vi "Main.vi"(11 "Module Admin":refnum<class "Delacor_lib_QMH_Module Admin.lvclass">) -> ()   [LabVIEW 2019, in "CONFIG .lvlib"]
doc: "This template is based off of the Queued Message Handler design pattern and the Queued Message Handler project template that ships with LabVIEW.\n\nThe main difference is that the queue is private to this module and communication between modules is performed via Broadcast and Request events.\n\nRequest events are wrapped in public API methods and are handled in the Event Handling Loop (EHL) of this VI. Any module can register for Broadcast events sent by this module. The EHL generates messages based on user interface actions.\n\nThe Message Handling Loop (MHL) processes messages generated by the EHL, or by other messages. The messages are string values, so new messages can be added easily to the Message Cases case structure in the MHL. Each message cluster can also provide an optional value for Message Data, which is a variant that can be converted to whatever message-specific data is required.\n_____\nBased on Delacor QMH Project Template 5.0.0.82."
uses:
  CONFIG .lvlib
  <vilib>/Delacor/Delacor QMH/Libraries/Module Admin_class/Delacor_lib_QMH_Module Admin.lvclass
  Module Data--cluster.ctl
  STOP HELPER LOOP CONFIG Argument--cluster.ctl
  <vilib>/Delacor/Delacor QMH/Libraries/Message Queue_class/Delacor_lib_QMH_Message Queue.lvclass/Delacor_lib_QMH_Message Queue.ctl
  Stop Argument--cluster.ctl
  <vilib>/Delacor/Delacor QMH/Libraries/Module Admin_class/Delacor_lib_QMH_Module Admin.lvclass/Delacor_lib_QMH_Module Admin.ctl
  CONFIG START HELPER LOOP Argument--cluster.ctl
  <vilib>/Utility/miscctls.llb/LVPointTypeDef.ctl
  <vilib>/Delacor/Delacor QMH/Libraries/Message Queue_class/Delacor_lib_QMH_Enqueue Message (Single).vi
  <vilib>/Delacor/Delacor QMH/Libraries/Module Admin_class/Delacor_lib_QMH_Get External Launch.vi
  <vilib>/Utility/error.llb/Error Cluster From Error Code.vi
  <vilib>/ErrorRing/Error Ring.xnode
  <vilib>/Delacor/Delacor QMH/Libraries/Message Queue_class/Delacor_lib_QMH_Message Queue.lvclass
panel:
  in  "Simulate MHL Error":bool
  in  "Simulate EHL Error":bool
  out "error out":errorcluster
  out "Status":string
  # "Other QMH Modules communicate with this Module via its Public API (wrappers for its Request Events).\n\nThis Module communicates with other Modules via its Broadcast Events.\nAny module that wants to get these messages, just registers for this module's Broadcast events."
  # "This template is for the Delacor Modified Queued Message Handler design pattern.\n\nSee the block diagram for more information on how to use this template."
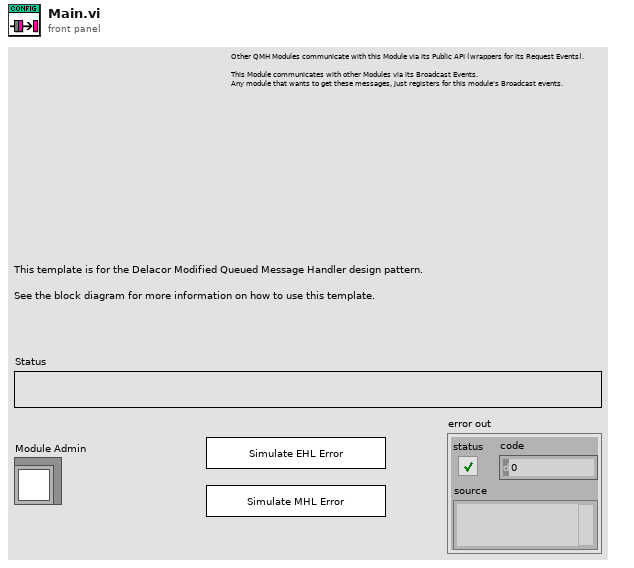
[diagram p1: front panel]
types:
  T1 = typedef "CONFIG .lvlib/Request Events--cluster.ctl" = cluster{"Stop Module":refnum<user-event>, "Show Panel":refnum<user-event>, "Hide Panel":refnum<user-event>, "Get Module Execution Status":refnum<user-event>, "Show Diagram":refnum<user-event>, "CONFIG START HELPER LOOP":refnum<user-event>, "STOP HELPER LOOP CONFIG":refnum<user-event>}
  T2 = typedef "CONFIG .lvlib/Module Data--cluster.ctl" = cluster{"Status":string}
  T3 = typedef "CONFIG .lvlib/STOP HELPER LOOP CONFIG Argument--cluster.ctl" = cluster{"Boolean":bool}
  T4 = enum32{"invalid lock state", "Not Locked", "Locked (No Password)", "Password-protected"}
  T5 = typedef "CONFIG .lvlib/Stop Argument--cluster.ctl" = cluster{"Origin":string, "Exit via Stop Module Req?":bool, "Wait for Module to stop?":bool}
  T6 = typedef "CONFIG .lvlib/CONFIG START HELPER LOOP Argument--cluster.ctl" = cluster{"DELAY TIMEOUT":i32}
  T7 = typedef "LVPointTypeDef.ctl" = cluster{"Horizontal":i16, "Vertical":i16}
  T8 = enum32{"Invalid", "Standard", "Closed", "Hidden", "Minimized", "Maximized"}
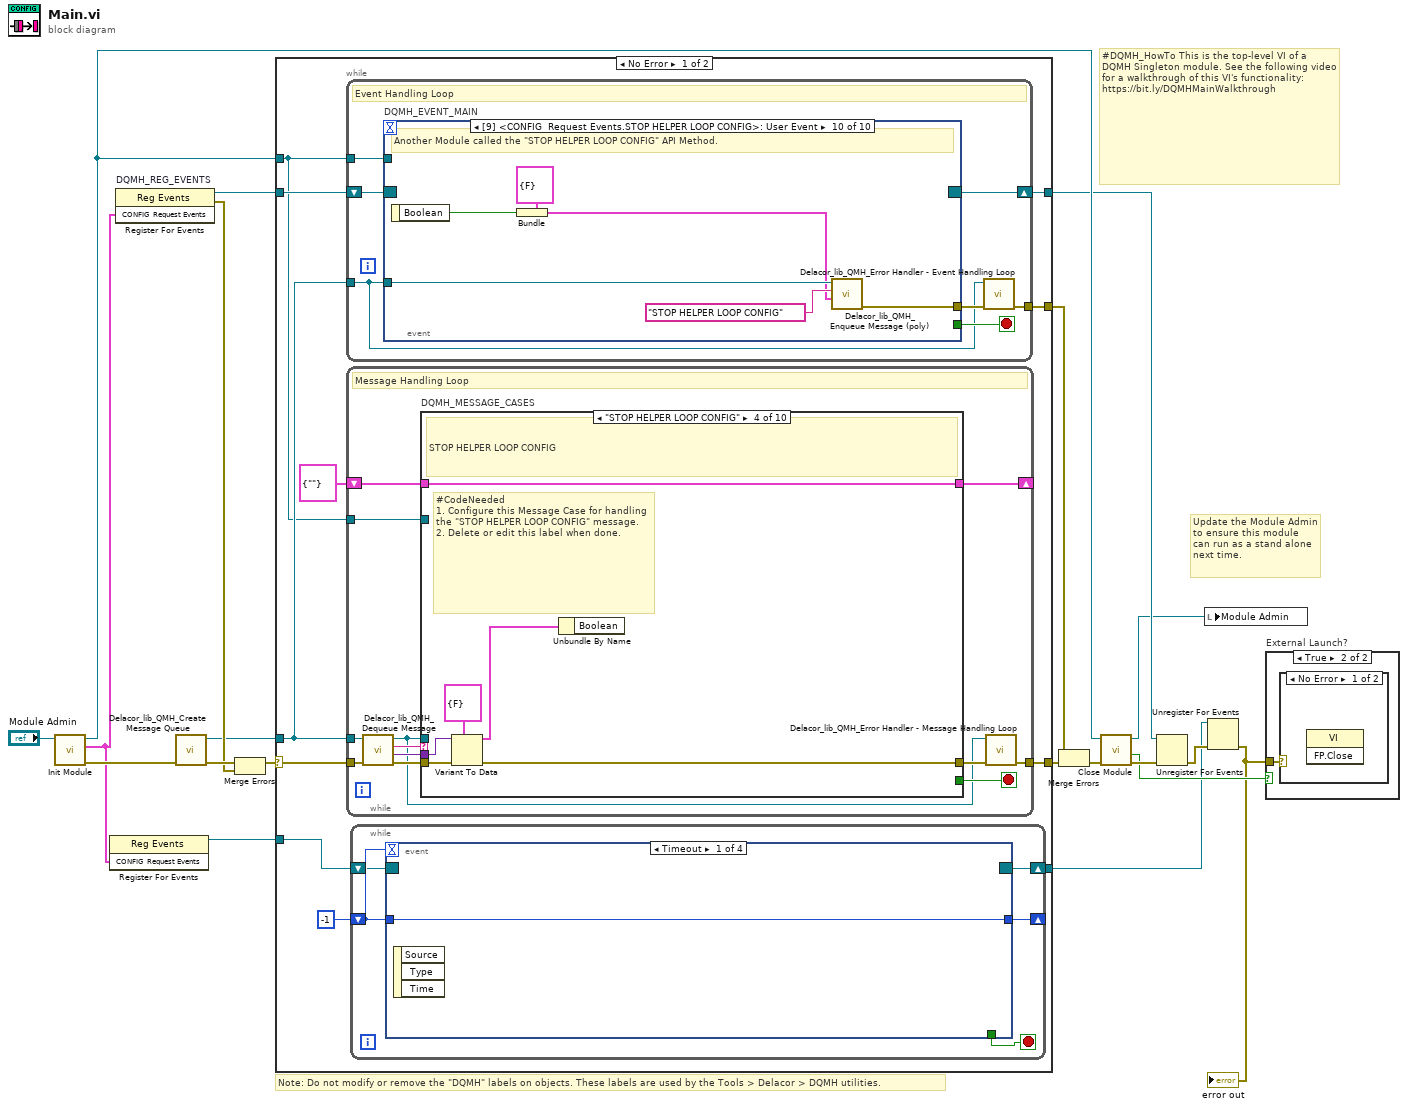
[diagram p0: block diagram]
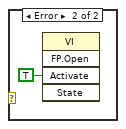
[diagram p3: hidden frame]
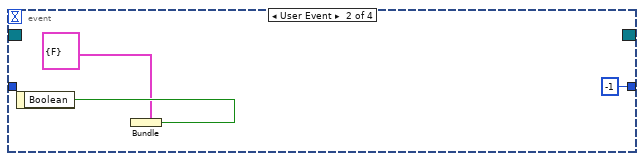
[diagram p4: hidden frame]
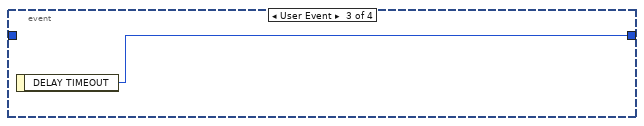
[diagram p5: hidden frame]
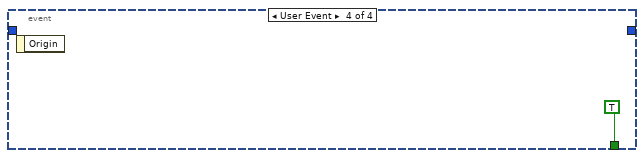
[diagram p6: hidden frame]
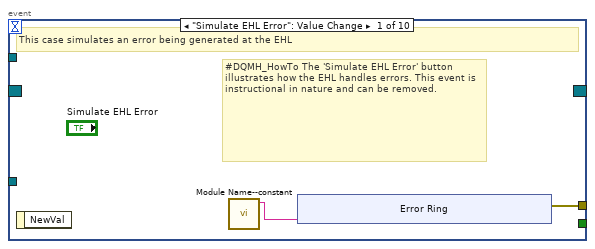
[diagram p7: hidden frame]
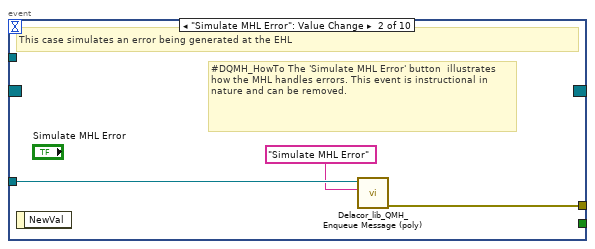
[diagram p8: hidden frame]
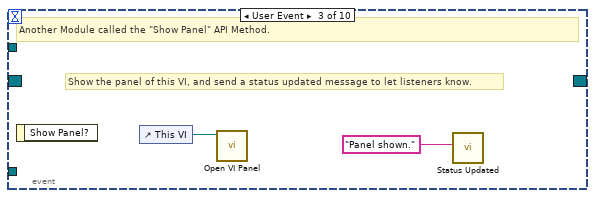
[diagram p9: hidden frame]
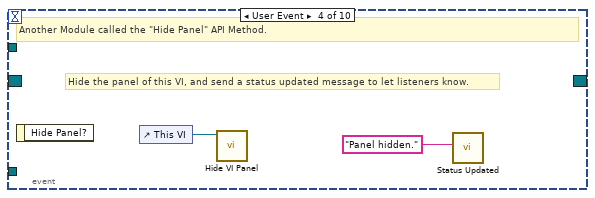
[diagram p10: hidden frame]
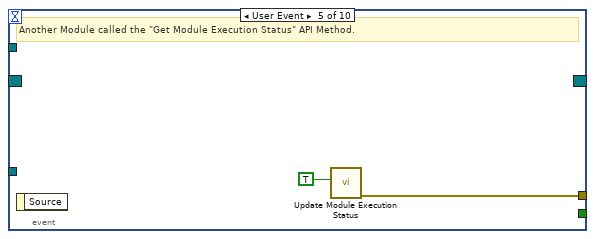
[diagram p11: hidden frame]
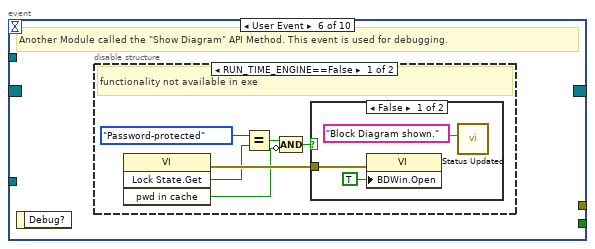
[diagram p12: hidden frame]
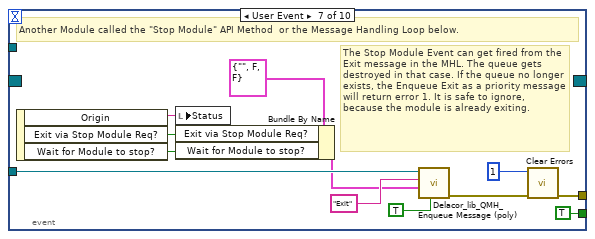
[diagram p15: hidden frame]
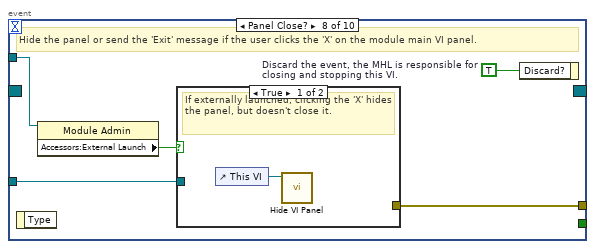
[diagram p16: hidden frame]
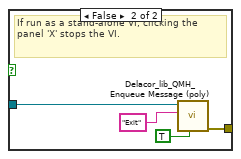
[diagram p17: hidden frame]
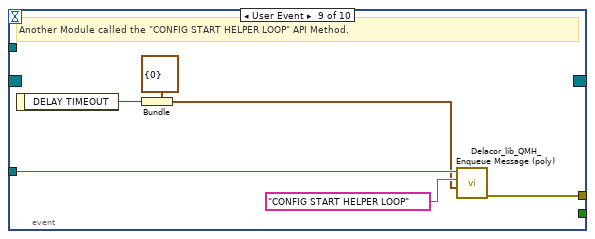
[diagram p18: hidden frame]
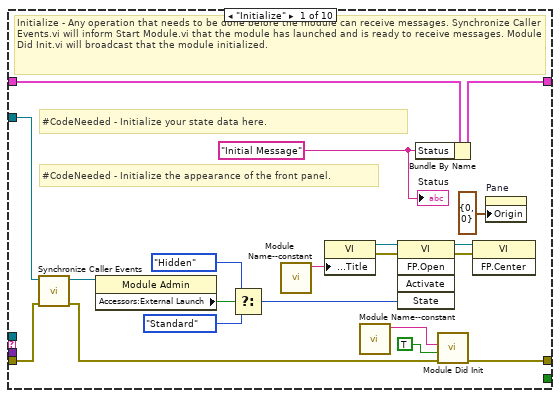
[diagram p19: hidden frame]
diagram:
  # "#DQMH_HowTo This is the top-level VI of a DQMH Singleton module. See the following video for a walkthrough of this VI's functionality: https://bit.ly/DQMHMainWalkthrough"
  # "Note: Do not modify or remove the \"DQMH\" labels on objects. These labels are used by the Tools > Delacor > DQMH utilities."
  # "Update the Module Admin to ensure this module can run as a stand alone next time."
  n1 = call "Init Module.vi"("Singleton Module Admin in"="Module Admin") -> ("error out"=w19:errorcluster, "CONFIG  Request Events"=w5:T1, "Singleton Module Admin out"=w12:refnum<class "Delacor_lib_QMH_Module Admin.lvclass">)  [unwired: 8 in]
  n2 = register-events(w5) -> (reference out=w4:refnum<event-registration>)  [unwired: 2 in, 1 out]
  n3 = register-events "DQMH_REG_EVENTS"(w5) -> (reference out=w10:refnum<event-registration>, error out=w13:errorcluster)  [unwired: 2 in]
  n4 = call <vilib>:"Delacor_lib_QMH_Create Message Queue.vi"("error in (no error)"=w19) -> ("error out"=w15:errorcluster, "Message Queue"=w9:refnum<class "Delacor_lib_QMH_Message Queue.lvclass">)  [unwired: 9 in]
  n5 = Merge Errors(w15, w13) -> (w14:errorcluster)
  n6 = case shown="No Error" w14 {
    selector: w14 -> [w29 w223]
    tunnel: [w31 w222] -> w20
    tunnel: [w28 w228] -> w11
    tunnel: w10 -> [w26 w228]
    tunnel: w9 -> [w25 w221]
    tunnel: [w30 _] -> w17
    tunnel: w12 -> [w24 w224]
    tunnel: w4 -> [w22 w220]
    tunnel: [w21 w220] -> w2
    frame No Error {
      n7 = while {
        tunnel: w25 -> [w43]
        shift-right: [w46] -> w28
        shift-left: w26 -> [w47]
        tunnel: [w48] -> w30
        tunnel: w24 -> [w44]
        stop <- w45 stop-if-true
        # "Event Handling Loop"
        n8 = event "DQMH_EVENT_MAIN" shown="[9] <CONFIG  Request Events.STOP HELPER LOOP CONFIG>: User Event" {
          selector: w47 -> [_ _ _ _ _ _ _ _ _ _]
          dyn-events: [_ _ _ _ _ _ _ _ _ _] -> w46
          timeout: _ -> [_ _ _ _ _ _ _ _ _ _]
          tunnel: [_ _ _ _ _ _ TRUE ("Discard?") _ _ _] -> w45
          tunnel: w43 -> [_ w60 _ _ _ _ w84 w91 w104 w110]
          tunnel: [w51 w61 _ _ w67 _ w87 w93 w99 w105] -> w49
          tunnel: w44 -> [_ _ _ _ _ _ _ w90 _ _]
          event "Simulate EHL Error": Value Change {
            # "#DQMH_HowTo The 'Simulate EHL Error' button  illustrates how the EHL handles errors. This event is instructional in nature and can be removed."
            # "This case simulates an error being generated at the EHL"
            n9 = event-data() -> ()  [unwired: 1 in, 1 out]
            n10 = call "Module Name--constant.vi"() -> ("Module Name"=w50:string)  [unwired: 11 in]
            n11 = xnode "Error Ring"("parameter 0"=w50) -> ("error out"=w51:errorcluster)
          }
          event "Simulate MHL Error": Value Change {
            # "#DQMH_HowTo The 'Simulate MHL Error' button  illustrates how the MHL handles errors. This event is instructional in nature and can be removed."
            # "This case simulates an error being generated at the EHL"
            n12 = event-data() -> ()  [unwired: 1 in, 1 out]
            n13 = call-poly <vilib>:"Delacor_lib_QMH_Enqueue Message (poly).vi"("Message"="Simulate MHL Error", "Message Queue in"=w60) -> ("error out"=w61:errorcluster)  [unwired: 8 in, 1 out]
          }
          event User Event {
            # "Show the panel of this VI, and send a status updated message to let listeners know."
            # "Another Module called the \"Show Panel\" API Method."
            n14 = event-data() -> ()  [unwired: 1 in, 1 out]
            n15 = control-ref of="This VI"() -> (w63:refnum<vi>)
            n16 = call "Open VI Panel.vi"("VI"=w63) -> ()  [unwired: 10 in, 1 out]
            n17 = call "Status Updated.vi"("Status"="Panel shown." ("format string")) -> ()  [unwired: 10 in, 1 out]
          }
          event User Event {
            # "Hide the panel of this VI, and send a status updated message to let listeners know."
            # "Another Module called the \"Hide Panel\" API Method."
            n18 = event-data() -> ()  [unwired: 1 in, 1 out]
            n19 = control-ref of="This VI"() -> (w65:refnum<vi>)
            n20 = call "Hide VI Panel.vi"("VI"=w65) -> ()  [unwired: 10 in, 1 out]
            n21 = call "Status Updated.vi"("Status"="Panel hidden." ("format string")) -> ()  [unwired: 10 in, 1 out]
          }
          event User Event {
            # "Another Module called the \"Get Module Execution Status\" API Method."
            n22 = event-data() -> ()  [unwired: 1 in, 1 out]
            n23 = call "Update Module Execution Status.vi"("Running?"=TRUE) -> ("error out"=w67:errorcluster)  [unwired: 10 in]
          }
          event User Event {
            # "Another Module called the \"Show Diagram\" API Method. This event is used for debugging."
            n24 = event-data() -> ()  [unwired: 1 in, 1 out]
            n25 = disable-structure shown="RUN_TIME_ENGINE==False" {
              frame condition #0 (active) {
                # "functionality not available in exe"
                n26 = invoke class="VI" method="Lock State.Get"() -> (error out=w73:errorcluster, "Get Lock State"=w72:T4, "pwd in cache"=w69:bool)  [unwired: 4 in, 1 out]
                n27 = Equal?(x=T4."Password-protected", y=w72) -> (x = y?=w70:bool)
                n28 = Compound Arithmetic op=AND(w70, invert w69) -> (w68:bool)
                n29 = case shown="False" w68 {
                  tunnel: w73 -> [w76 _]
                  frame False {
                    n30 = property class="VI"(error in=w76, "BDWin.Open"=TRUE ("Block Diagram Window:Open")) -> ()  [unwired: 1 in, 2 out]
                    n31 = call "Status Updated.vi"("Status"="Block Diagram shown." ("format string")) -> ()  [unwired: 10 in, 1 out]
                  }
                  frame True {
                    # "Password-protected VI, and the password is not in the cache. Do not show the diagram."
                  }
                }
              }
              frame condition #1 {
              }
            }
          }
          event User Event {
            # "The Stop Module Event can get fired from the Exit message in the MHL. The queue gets destroyed in that case. If the queue no longer exists, the Enqueue Exit as a priority message will return error 1. It is safe to ignore, because the module is already exiting."
            # "Another Module called the \"Stop Module\" API Method  or the Message Handling Loop below."
            n32 = event-data() -> ("Origin"=w83:string, "Exit via Stop Module Req?"=w79:bool, "Wait for Module to stop?"=w78:bool)  [unwired: 1 in]
            n33 = local write "Status"(w83) -> ()
            n34 = Bundle By Name(cluster=T5 {"Origin"="", "Exit via Stop Module Req?"=FALSE, "Wait for Module to stop?"=FALSE} ("Stop Argument"), "Exit via Stop Module Req?"=w79, "Wait for Module to stop?"=w78) -> (w77:T5)
            n35 = call-poly <vilib>:"Delacor_lib_QMH_Enqueue Message (poly).vi"("Priority Message? (F)"=TRUE, "Message Data"=w77, "Message"="Exit", "Message Queue in"=w84) -> ("error out"=w88:errorcluster)  [unwired: 6 in, 1 out]
            n36 = call <vilib>:"Clear Errors.vi"("error in (no error)"=w88, "specific error code to clear (0: all)"=1) -> ("error out"=w87:errorcluster)  [unwired: 4 in, 1 out]
          }
          event Panel Close? {
            w92 = TRUE  # Discard the event, the MHL is responsible for closing and stopping this VI.
            # "Hide the panel or send the 'Exit' message if the user clicks the 'X' on the module main VI panel."
            n37 = event-data() -> ()  [unwired: 1 in, 1 out]
            n38 = property class="Module Admin"(reference=w90) -> ("Accessors:External Launch"=w89:bool)  [unwired: 1 in, 2 out]
            n39 = case shown="True" w89 {
              tunnel: w91 -> [_ w97]
              tunnel: [_ w98] -> w93
              frame True {
                # "If externally launched, clicking the 'X' hides the panel, but doesn't close it."
                n40 = control-ref of="This VI"() -> (w94:refnum<vi>)
                n41 = call "Hide VI Panel.vi"("VI"=w94) -> ()  [unwired: 10 in, 1 out]
              }
              frame False {
                # "If run as a stand-alone VI, clicking the panel 'X' stops the VI."
                n42 = call-poly <vilib>:"Delacor_lib_QMH_Enqueue Message (poly).vi"("Priority Message? (F)"=TRUE, "Message"="Exit", "Message Queue in"=w97) -> ("error out"=w98:errorcluster)  [unwired: 7 in, 1 out]
              }
            }
            n43 = event-data("Discard?"=w92) -> ()  [unwired: 1 in, 1 out]
          }
          event User Event {
            # "Another Module called the \"CONFIG START HELPER LOOP\" API Method."
            n44 = event-data() -> ("DELAY TIMEOUT"=w100:i32)  [unwired: 1 in]
            n45 = Bundle(cluster=T6 {"DELAY TIMEOUT"=0} ("CONFIG START HELPER LOOP Argument"), "DELAY TIMEOUT"=w100) -> (w101:T6)
            n46 = call-poly <vilib>:"Delacor_lib_QMH_Enqueue Message (poly).vi"("Message Data"=w101, "Message"="CONFIG START HELPER LOOP", "Message Queue in"=w104) -> ("error out"=w99:errorcluster)  [unwired: 7 in, 1 out]
          }
          event User Event {
            # "Another Module called the \"STOP HELPER LOOP CONFIG\" API Method."
            n47 = event-data() -> ("Boolean"=w106:bool)  [unwired: 1 in]
            n48 = Bundle(cluster=T3 {"Boolean"=FALSE} ("STOP HELPER LOOP CONFIG Argument"), "Boolean"=w106) -> (w107:T3)
            n49 = call-poly <vilib>:"Delacor_lib_QMH_Enqueue Message (poly).vi"("Message Data"=w107, "Message"="STOP HELPER LOOP CONFIG", "Message Queue in"=w110) -> ("error out"=w105:errorcluster)  [unwired: 7 in, 1 out]
          }
        }
        n50 = call-dynamic "Delacor_lib_QMH_Error Handler - Event Handling Loop.vi"("error in (no error)"=w49, "Message Queue in"=w43) -> ("dup error in"=w48:errorcluster)  [unwired: 8 in, 1 out]
      }
      n51 = while {
        tunnel: w25 -> [w113]
        shift-right: [w117] -> _
        shift-left: T2 {"Status"=""} ("Data Cluster") -> [w118]
        tunnel: w29 -> [w121]
        tunnel: [w119] -> w31
        tunnel: w24 -> [w111]
        stop <- w116 stop-if-true
        # "Message Handling Loop"
        n52 = call-dynamic "Delacor_lib_QMH_Dequeue Message.vi"("error in (no error)"=w121, "Message Queue in"=w113) -> ("error out"=w120:errorcluster, "Message Data"=w114:variant, "Message"=w115:string, "Message Queue out"=w112:refnum<class "Delacor_lib_QMH_Message Queue.lvclass">)  [unwired: 6 in]
        n53 = case "DQMH_MESSAGE_CASES" shown="\"STOP HELPER LOOP CONFIG\"" w115 {
          selector: w115 -> [_ _ _ _ _ _ _ _ _ w207]
          tunnel: w112 -> [_ _ _ _ _ _ _ w177 w199 _]
          tunnel: w120 -> [w140 w144 w150 w156 w159 w161 w166 w184 w205 w209]
          tunnel: [w138 w144 w148 w154 w158 w161 w165 w180 w202 w210] -> w122
          tunnel: w118 -> [w129 w143 w149 w155 w157 w160 w163 w179 w198 w208]
          tunnel: [w128 w143 w149 w155 w157 w160 w163 w179 w198 w208] -> w117
          tunnel: [_ _ _ _ _ _ _ _ w197 _] -> w116
          tunnel: w114 -> [_ _ w147 w153 _ _ _ w178 w196 _]
          tunnel: w111 -> [w130 _ _ _ _ _ _ w176 w191 _]
          frame "Initialize" {
            w123 = "Initial Message" ("Initial Message")
            # "#CodeNeeded - Initialize the appearance of the front panel."
            # "#CodeNeeded - Initialize your state data here."
            # "Initialize - Any operation that needs to be done before the module can receive messages. Synchronize Caller Events.vi will inform Start Module.vi that the module has launched and is ready to receive messages. Module Did Init.vi will broadcast that the module initialized."
            n54 = call "Synchronize Caller Events.vi"("error in (no error)"=w140, "Singleton Module Admin in"=w130) -> ("error out"=w139:errorcluster, "Singleton Module Admin out"=w125:refnum<class "Delacor_lib_QMH_Module Admin.lvclass">)  [unwired: 8 in]
            n55 = property class="Module Admin"(reference=w125) -> ("Accessors:External Launch"=w134:bool)  [unwired: 1 in, 2 out]
            n56 = Select(t=T8."Hidden" ("State"), s=w134, f=T8."Standard" ("State")) -> (s? t:f=w131:T8)
            n57 = call "Module Name--constant.vi"() -> ("Module Name"=w137:string)  [unwired: 11 in]
            n58 = property class="VI"("Front Panel.Title"=w137) -> (reference out=w136:refnum<vi>, error out=w142:errorcluster)  [unwired: 2 in]
            n59 = call "Module Name--constant.vi"() -> ("Module Name"=w126:string)  [unwired: 11 in]
            n60 = invoke class="VI" method="FP.Open"(reference=w136, error in=w142, "State"=w131) -> (reference out=w135:refnum<vi>, error out=w141:errorcluster)  [unwired: 2 in, 3 out]
            n61 = Bundle By Name(cluster=w129, "Status"=w123) -> (w128:T2)
            n62 = call "Module Did Init.vi"("error in (no error)"=w139, "Initialized?"=TRUE, "Origin"=w126) -> ("error out"=w138:errorcluster)  [unwired: 8 in]
            n63 = invoke class="VI" method="FP.Center"(reference=w135, error in=w141) -> ()  [unwired: 1 in, 3 out]
            n64 = property on="Pane" class="Pane"("Origin"=T7 {"Horizontal"=0, "Vertical"=0}) -> ()  [unwired: 2 in, 2 out]
            "Status" <- w123
          }
          frame "--- Module Specific ---" {
            # "Separator -- The following cases handle messages specific to this Module."
          }
          frame "CONFIG START HELPER LOOP" {
            # "#CodeNeeded\n1. Configure this Message Case for handling the \"CONFIG START HELPER LOOP\" message.\n2. Delete or edit this label when done."
            # "CONFIG START HELPER LOOP"
            n65 = Variant To Data(error in=w150, type=T6 {"DELAY TIMEOUT"=0} ("CONFIG START HELPER LOOP Argument"), Variant=w147) -> (data=w145:T6, error out=w148:errorcluster)
            n66 = Unbundle By Name(w145) -> ()  [unwired: 1 out]
          }
          frame "STOP HELPER LOOP CONFIG" {
            # "#CodeNeeded\n1. Configure this Message Case for handling the \"STOP HELPER LOOP CONFIG\" message.\n2. Delete or edit this label when done."
            # "STOP HELPER LOOP CONFIG"
            n67 = Variant To Data(error in=w156, type=T3 {"Boolean"=FALSE} ("STOP HELPER LOOP CONFIG Argument"), Variant=w153) -> (data=w151:T3, error out=w154:errorcluster)
            n68 = Unbundle By Name(w151) -> ()  [unwired: 1 out]
          }
          frame "---Copy This Frame---" {
            # "Duplicate this frame when creating new messages.  Change this comment in the duplicated frame to describe this message."
            n69 = Merge Errors(w159) -> (w158:errorcluster)
          }
          frame "--- Exit and Error Handling---" {
            # "Separator - The following cases handle errors and exit messages."
          }
          frame "Simulate MHL Error" {
            # "#DQMH_HowTo The 'Simulate MHL Error' button  illustrates how the MHL handles errors. This event is instructional in nature and can be removed."
            # "Simulate an error occurring at the MHL"
            n70 = call "Module Name--constant.vi"() -> ("Module Name"=w162:string)  [unwired: 11 in]
            n71 = xnode "Error Ring"("parameter 0"=w162) -> ("error out"=w164:errorcluster)
            n72 = Merge Errors(w166, w164) -> (w165:errorcluster)
          }
          frame "Error" {
            # "#CodeRecommended - If you ever change the name of this \"Error\" message, you'll need to update the name in the Check Loop Error.vi as well."
            # "#CodeRecommended - If the module is running in standalone mode (External Launch = FALSE), this code will pop up an error dialog and call the 'Exit' message if an error occurs. Add more fine-grained error handling here."
            # "Error - Check the error message data and respond accordingly. This message is sent by the \"Error Handler\" VIs at the end of each loop in this application."
            n73 = property class="Module Admin"(reference=w176) -> ("Accessors:External Launch"=w175:bool)  [unwired: 1 in, 2 out]
            n74 = Variant To Data(error in=w184, type=errorcluster {"status"=FALSE, "code"=0, "source"=""} ("error constant"), Variant=w178) -> (data=w185:errorcluster, error out=w182:errorcluster)
            n75 = call "Module Name--constant.vi"() -> ("Module Name"=w174:string)  [unwired: 11 in]
            n76 = call "Error Reported.vi"("Additional Information"=w174, "Error"=w185) -> ()  [unwired: 9 in, 1 out]
            n77 = case shown="False" w175 {
              tunnel: [w190 _] -> w181
              tunnel: w177 -> [w188 _]
              tunnel: w185 -> [w189 _]
              frame False {
                # "If the module is running standalone, then pop up an error dialog and call the \"Exit\" message."
                n78 = call <vilib>:"Simple Error Handler.vi"("error in (no error)"=w189) -> ()  [unwired: 4 in, 5 out]
                n79 = call-poly <vilib>:"Delacor_lib_QMH_Enqueue Message (poly).vi"("Priority Message? (F)"=TRUE, "Message"="Exit", "Message Queue in"=w188) -> ("error out"=w190:errorcluster)  [unwired: 7 in, 1 out]
              }
              frame True {
                # "If the module was launched externally, calling the Error Reported broadcast VI is the only action performed by the \"Error\" message. The module's caller can then process the error appropriately."
              }
            }
            n80 = Merge Errors(w182, w181) -> (w180:errorcluster)
            n81 = local write "error out"(w180) -> ()
          }
          frame "Exit" {
            w195 = 91  # 91: not all Exit messages will have an argument
            w197 = TRUE  # Stop the VI
            # "Release the message queue reference"
            # "#CodeNeeded - Add any required cleanup code here"
            # "Exit - Exit the application."
            n82 = Variant To Data(error in=w205, type=T5 {"Origin"="", "Exit via Stop Module Req?"=FALSE, "Wait for Module to stop?"=FALSE} ("Stop Argument"), Variant=w196) -> (data=w193:T5, error out=w201:errorcluster)
            n83 = call <vilib>:"Clear Errors.vi"("error in (no error)"=w201, "specific error code to clear (0: all)"=w195) -> ("error out"=w204:errorcluster)  [unwired: 4 in, 1 out]
            n84 = control-ref of="This VI"() -> (w192:refnum<vi>)
            n85 = call-dynamic "Delacor_lib_QMH_Release Message Queue.vi"("error in (no error)"=w204, "Message Queue"=w199) -> ("error out"=w203:errorcluster)  [unwired: 9 in]
            n86 = call "Handle Exit.vi"("Stop Argument"=w193, "Admin in"=w191, "VI reference"=w192) -> ("error out"=w200:errorcluster)  [unwired: 7 in, 1 out]
            n87 = Merge Errors(w203, w200) -> (w202:errorcluster)
          }
          frame Default {
            # "'Default' case only runs if there is a message that isn't defined in any of the other cases.  Output a programming error."
            n88 = call "Module Name--constant.vi"() -> ("Module Name"=w206:string)  [unwired: 11 in]
            n89 = xnode "Error Ring"("parameter 0"=w207, "parameter 1"=w206) -> ("error out"=w211:errorcluster)
            n90 = Merge Errors(w209, w211) -> (w210:errorcluster)
          }
        }
        n91 = call-dynamic "Delacor_lib_QMH_Error Handler - Message Handling Loop.vi"("error in (no error)"=w122, "Message Queue in"=w112) -> ("dup error in"=w119:errorcluster)  [unwired: 8 in, 1 out]
      }
      n92 = while {
        shift-right: [w34] -> w21
        shift-left: w22 -> [w35]
        shift-right: [w33] -> _
        shift-left: -1 ("DELAY TIMEOUT") -> [w36]
        stop <- w32 stop-if-true
        n93 = event shown="[0] Timeout" {
          selector: w35 -> [_ _ _ _]
          dyn-events: [_ _ _ _] -> w34
          timeout: w36 -> [_ _ _ _]
          tunnel: [_ _ _ TRUE ("stop")] -> w32
          tunnel: [w37 -1 ("DELAY TIMEOUT") w41 _] -> w33
          tunnel: w36 -> [w37 _ _ _]
          event Timeout {
            n94 = event-data() -> ()  [unwired: 1 in, 3 out]
          }
          event User Event {
            n95 = event-data() -> ("Boolean"=w40:bool)  [unwired: 1 in]
            n96 = Bundle(cluster=T3 {"Boolean"=FALSE} ("STOP HELPER LOOP CONFIG Argument"), "Boolean"=w40) -> ()  [unwired: 1 out]
          }
          event User Event {
            n97 = event-data() -> ("DELAY TIMEOUT"=w41:i32)  [unwired: 1 in]
          }
          event User Event {
            n98 = event-data() -> ()  [unwired: 1 in, 1 out]
          }
        }
      }
    }
    frame Error {
      # "Synchronize Caller Events.vi will inform Start Module.vi that the module has launched and will let the code calling Start Module.vi register for broadcasts and would permit the caller receive the broadcast that an error occurred at launch time."
      n99 = call-dynamic "Delacor_lib_QMH_Release Message Queue.vi"("error in (no error)"=w223, "Message Queue"=w221) -> ("error out"=w222:errorcluster)  [unwired: 9 in]
      n100 = call "Synchronize Caller Events.vi"("Singleton Module Admin in"=w224) -> ("error out"=w229:errorcluster)  [unwired: 9 in, 1 out]
      n101 = call "Module Name--constant.vi"() -> ("Module Name"=w227:string)  [unwired: 11 in]
      n102 = Format Into String(format string="An error occurred during initialization. %s is no longer running.", w227) -> (resulting string=w225:string)  [unwired: 2 in, 1 out]
      n103 = Merge Errors(w222, w229) -> (w230:errorcluster)
      n104 = call "Error Reported.vi"("Additional Information"=w225, "Error"=w230) -> ()  [unwired: 9 in, 1 out]
    }
  }
  n105 = Merge Errors(w17, w20) -> (w16:errorcluster)
  n106 = call "Close Module.vi"("error in (no error)"=w16, "Module Admin in"=w12) -> ("error out"=w18:errorcluster, "External Launch"=w6:bool, "Module Admin out"=w7:refnum<class "Delacor_lib_QMH_Module Admin.lvclass">)  [unwired: 7 in]
  n107 = Unregister For Events(event registration refnum=w11, error in=w18) -> (error out=w3:errorcluster)
  n108 = local write "Module Admin"(w7) -> ()
  n109 = Unregister For Events(event registration refnum=w2, error in=w3) -> (error out=w1:errorcluster)
  "error out" <- w1
  n110 = case "External Launch?" shown="True" w6 {
    tunnel: w1 -> [_ w231]
    frame False {
    }
    frame True {
      n111 = case shown="No Error" w231 {
        frame No Error {
          n112 = invoke class="VI" method="FP.Close"() -> ()  [unwired: 3 in, 3 out]
        }
        frame Error {
          n113 = invoke class="VI" method="FP.Open"("Activate"=TRUE ("Activate?")) -> ()  [unwired: 4 in, 5 out]
        }
      }
    }
  }
